vi "PH_gentec_M-Link.PC Write PSDB.vi"(0 "i ref in":refnum<vi>, 5 "error IO":errorcluster) -> (14 "i ref out":refnum<vi>, 19 "error out":errorcluster)   [LabVIEW 2014, in "PH_gentec_M-Link.lvlib"]
doc: "This is the proc case which writes data to the PHELIX shot data base."
uses:
  PH_gentec_M-Link.lvlib
  non_GPL/instr.lib/gentec-M-LINK/Driver/Type Defs/gentec-M-Link.Trigger Source.ctl
  non_GPL/instr.lib/gentec-M-LINK/gentec-M-Link - Driver.lvlib
  PH_PSDBWriter/PH_PSDBWriter.lvlib
  PH_Powermeter_BaseClass/PH_Powermeter_BaseClass.lvlib
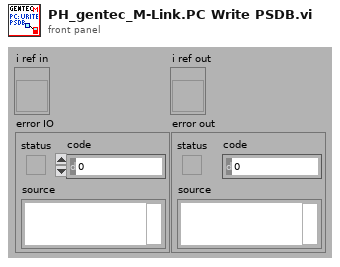
[diagram p1: front panel]
types:
  T1 = typedef "gentec-M-Link - Driver.lvlib/gentec-M-Link.Trigger Source.ctl" = u16
  T2 = typedef "PH_Powermeter_BaseClass.lvlib/PH_Powermeter_BaseClass.i attribute.ctl" = cluster{"GUI References":T3, "Connection":T4, "Head Attributes":T6, "VISA resource":refnum<visa-resource-name>, "Energy":T7, "Service ID Energy":i32, "Wanted Settings":T8, "Current Settings":T8}
  T3 = typedef "PH_Powermeter_BaseClass.lvlib/PH_Powermeter_BaseClass.GUI Refs.ctl" = cluster{"Head Attributes":refnum<vi>, "Energy":refnum<vi>, "Connection":refnum<vi>, "VISA Resource":refnum<vi>, "Energy evolution":refnum<vi>, "Scaling Factor":refnum<vi>, "Range":refnum<vi>, "Wavelength":refnum<vi>, "Trigger Level":refnum<vi>, "Wanted Settings":refnum<vi>, "Current Settings":refnum<vi>}
  T4 = typedef "PH_Powermeter_BaseClass.lvlib/PH_Powermeter_BaseClass.Connection.ctl" = cluster{"failed checks":i8, "Timeout":bool, "Data read":string, "Failure":bool, "Error":bool, "State":T5}
  T5 = typedef "PH_Powermeter_BaseClass.lvlib/PH_Powermeter_BaseClass.State.ctl" = enum32{"off", "operating", "opened", "checked", "connected", "Sets to change", "running"}
  T6 = typedef "PH_Powermeter_BaseClass.lvlib/PH_Powermeter_BaseClass.Head Attributes.ctl" = cluster{"Instrument Type":string, "Head Version":string, "Head Name":string, "Serial Number":string, "Firmware":string, "Sensor Type":string, "MinimumRange":u32, "Maximum Range":u32, "Min Wavelength":i32, "Max Wavelength":i32}
  T7 = typedef "PH_Powermeter_BaseClass.lvlib/PH_Powermeter_BaseClass.Energy.ctl" = cluster{"current Value":dbl, "unscaled":dbl, "Scaling Factor":dbl}
  T8 = typedef "PH_Powermeter_BaseClass.lvlib/PH_gentec_BaseClass.Head Settings.ctl" = cluster{"Trigger Level":dbl, "Wavelength":u32, "Range":u32}
  T9 = typedef "PH_gentec_M-Link.lvlib/PH_gentec_M-Link.i attribute.ctl" = cluster{"GUI References":cluster{"Wanted Head Settings":refnum<vi>, "Current Head Settings":refnum<vi>, "Set Auto Range":refnum<vi>, "Trigger Polarity":refnum<vi>, "Trigger Source":refnum<vi>, "Waveform Averages":refnum<vi>, "Continuous":refnum<vi>, "get one Value":refnum<vi>}, "Wanted Head Settings":T10, "Current Head Settings":T10}
  T10 = typedef "PH_gentec_M-Link.lvlib/PH_gentec_M-Link.Head Settings.ctl" = cluster{"Measurement Mode":T11, "Enable Anticipation":bool, "Set Auto Range":bool, "Block Signal":bool, "Set Head Attenuator":bool, "Enable SSE":bool, "Trigger Polarity":T12, "Trigger Source":T1, "Waveform Averages":T13, "Set Zero":i32, "Current Measurement":i32, "Start Data Flow":bool}
  T11 = typedef "gentec-M-Link - Driver.lvlib/gentec-M-Link.Measurement Mode.ctl" = u16
  T12 = typedef "gentec-M-Link - Driver.lvlib/gentec-M-Link.Trigger Polarity.ctl" = u16
  T13 = typedef "gentec-M-Link - Driver.lvlib/gentec-M-Link.Waveform Averages.ctl" = u16
  T14 = typedef "PH_PSDBWriter.lvlib/PH_PSDBWriter.Numeric dataset.ctl" = cluster{"name":string, "data":dbl, "unit":string}
  T15 = typedef "PH_PSDBWriter.lvlib/PH_PSDBWriter.String dataset.ctl" = cluster{"name":string, "data":string, "unit":string}
  T16 = typedef "PH_PSDBWriter.lvlib/PH_PSDBWriter.PSDB Dataset.ctl" = cluster{"Version":i32, "2D data Input":T17[], "Boolean Input":T19[], "Image Input":T20[], "Numeric Input":T14[], "String Input":T15[]}
  T17 = typedef "PH_PSDBWriter.lvlib/PH_PSDBWriter.2D dataset.ctl" = cluster{"name":string, "data":dbl[][], "axis description":T18}
  T18 = typedef "PSDB.lvlib/PSDB_AxisDescription.ctl" = cluster{"x axis label":string, "y axis label":string, "x axis unit":string, "y axis unit":string}
  T19 = typedef "PH_PSDBWriter.lvlib/PH_PSDBWriter.Boolean dataset.ctl" = cluster{"name":string, "data":bool, "unit":string}
  T20 = typedef "PH_PSDBWriter.lvlib/PH_PSDBWriter.Image dataset.ctl" = cluster{"name":string, "data":T21, "unit":string}
  T21 = typedef "IMAQ Image.ctl" = refnum<image>
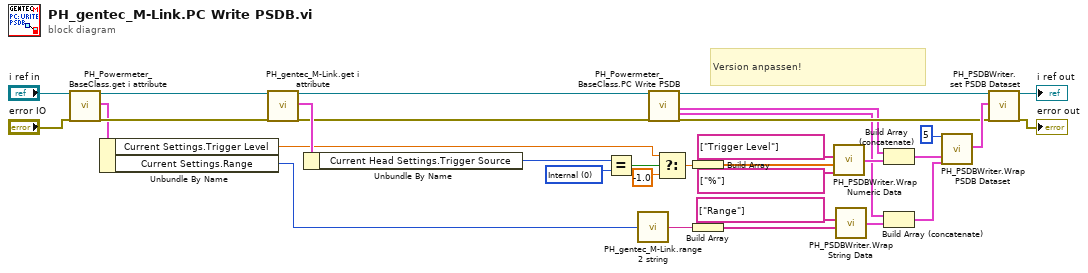
[diagram p0: block diagram]
diagram:
  w30 = T1 0 items=["Internal", "External"] ("Current Head Settings.Trigger Source")
  # "Version anpassen!"
  n1 = call "PH_Powermeter_BaseClass.get i attribute.vi"("i ref in"="i ref in", "error in (no error)"="error IO") -> ("i ref out"=w5:refnum<vi>, "i attribute"=w3:T2, "error out"=w4:errorcluster)  [unwired: 15 in]
  n2 = Unbundle By Name(w3) -> ("Current Settings.Trigger Level"=w2:dbl, "Current Settings.Range"=w1:u32)
  n3 = call "PH_gentec_M-Link.get i attribute.vi"("i ref in"=w5, "error in (no error)"=w4) -> ("i ref out"=w25:refnum<vi>, "i attribute"=w32:T9, "error out"=w7:errorcluster)  [unwired: 15 in]
  n4 = Unbundle By Name(w32) -> ("Current Head Settings.Trigger Source"=w31:T1)
  n5 = Equal?(x=w31, y=w30) -> (x = y?=w29:bool)
  n6 = call "PH_gentec_M-Link.range 2 string.vi"("Range"=w1) -> ("Range as string"=w8:string)
  n7 = call "PH_Powermeter_BaseClass.PC Write PSDB.vi"("i ref in"=w25, "error IO"=w7) -> ("i ref out"=w14:refnum<vi>, "PSDB Numeric Data Array"=w10:T14[], "PSDB String Data Array"=w9:T15[], "error out"=w13:errorcluster)  [unwired: 14 in]
  n8 = Select(t=w2, s=w29, f=-1.0) -> (s? t:f=w28:dbl)
  n9 = Build Array(w28) -> (w16:dbl[])
  n10 = Build Array(w8) -> (w18:string[])
  n11 = call "PH_PSDBWriter.Wrap Numeric Data.vi"("Unit Array"=string[] ["%"], "Data Array"=w16, "Name Array"=string[] ["Trigger Level"]) -> ("PSDB Numeric Data Array"=w23:T14[])  [unwired: 1 in]
  n12 = call "PH_PSDBWriter.Wrap String Data.vi"("Data Array"=w18, "Name Array"=string[] ["Range"]) -> ("PSDB String Data Array"=w22:T15[])  [unwired: 2 in]
  n13 = Build Array (concatenate)(w10, w23) -> (w12:T14[])
  n14 = Build Array (concatenate)(w9, w22) -> (w11:T15[])
  n15 = call "PH_PSDBWriter.Wrap PSDB Dataset.vi"("Version"=5, "Numeric Input"=w12, "String Input"=w11) -> ("PSDB Dataset"=w20:T16)  [unwired: 16 in]
  n16 = call "PH_PSDBWriter.set PSDB Dataset.vi"("VI in"=w14, "PSDB Dataset"=w20, "error in (no error)"=w13) -> ("VI out"=→"i ref out":refnum<vi>, "error out"=→"error out":errorcluster)  [unwired: 15 in]
